vi "PWRVT.vi"() -> ()   [LabVIEW 2017]
uses:
  FcutionVI/Modbus function.ctl
  dll/LabVIEW_CSLib.dll
  dll/Modbus.dll
panel:
  in  "Data type":enum16{"Raw", "OA"}(ring)
  out "SN":string
  out "Acc RMS":u16[](array[numeric])
  out "Stop Time":timestamp
  in  "stop":bool
  out "Waveform Chart":dbl[][](graph)=[[0.0015869140625, -0.000732421875, -0.001220703125], [0.0008544921875, -0.0009765625, 0.000244140625], [0.0006103515625, -0.001220703125, 0.001220703125], [0.0015869140625, -0.0006103515625, 0.00048828125], [0.001953125, 0.0, -0.00048828125], [0.0009765625, 0.0, -0.000732421875], [0.0010986328125, -0.000244140625, -0.0006103515625], [0.0020751953125, 0.000244140625, 0.0], [0.002197265625, 0.001220703125, 0.0006103515625], [0.0020751953125, 0.0009765625, -0.000244140625], [0.0020751953125, 0.0, -0.0018310546875], [0.0013427734375, 0.0, -0.001708984375], [0.00048828125, 0.0001220703125, -0.0008544921875], [0.0009765625, -0.000244140625, -0.0010986328125], [0.0009765625, -0.0008544921875, -0.00146484375], [-0.0003662109375, -0.0003662109375, -0.0003662109375], [-0.0010986328125, 0.0, 0.0001220703125], [-0.0003662109375, -0.000244140625, -0.0008544921875], [-0.0006103515625, -0.000244140625, -0.001708984375], [-0.00146484375, 0.0010986328125, 0.0], [-0.000732421875, 0.001953125, 0.002685546875], [0.000244140625, 0.0010986328125, 0.0037841796875], [0.0, 0.0003662109375, 0.002197265625], [-0.0006103515625, 0.0006103515625, -0.0006103515625]]
  out "Modbus Function":T1
  out "Data Length 抓資料後的剩餘長度":u16(graph)
  in  "DAQ Interval (ms)":u32
  in  "SlaveID":u8=1
  out "error out":errorcluster
  in  "stopBits":i32(ring)=1 items=["None", "One", "Two", "OnePointFive"]
  in  "dataBits":i32=8
  in  "parity":i32(ring) items=["None", "Odd", "Even", "Mark", "Space"]
  in  "baudRate":i32=3000000
  in  "VISA resource name":refnum<visa-resource-name>
  # "x"
  # "y"
  # "z"
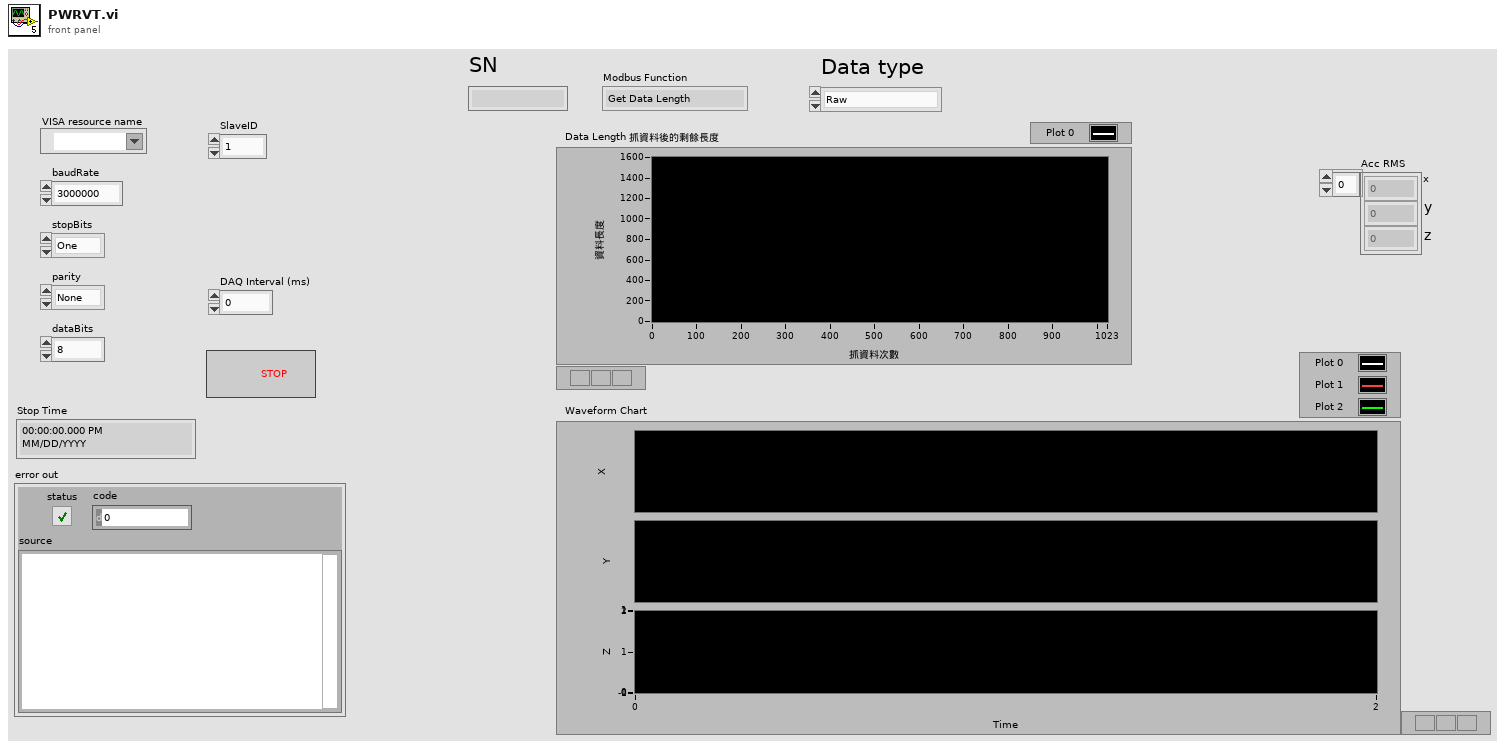
[diagram p1: front panel]
types:
  T1 = typedef "Modbus function.ctl" = enum16{"Get Data Length", "Normal Mode", "Bulk Mode"}
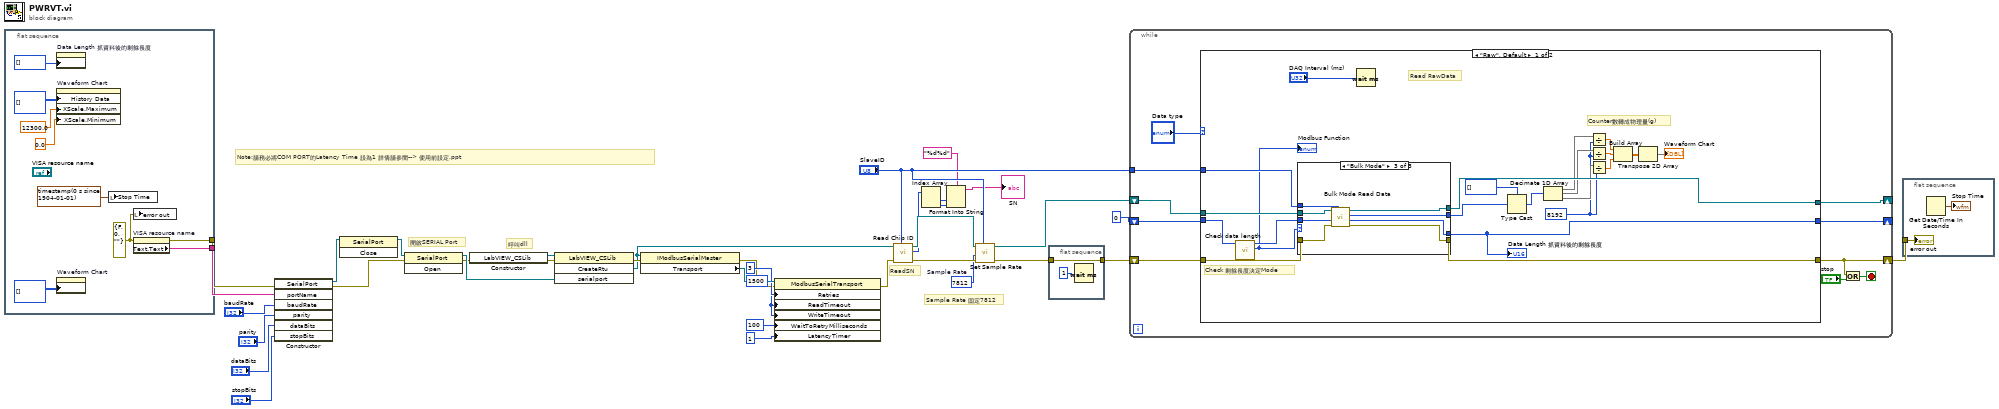
[diagram p0: block diagram]
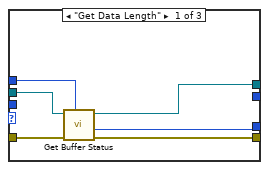
[diagram p2: hidden frame]
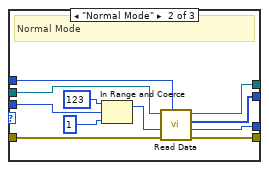
[diagram p3: hidden frame]
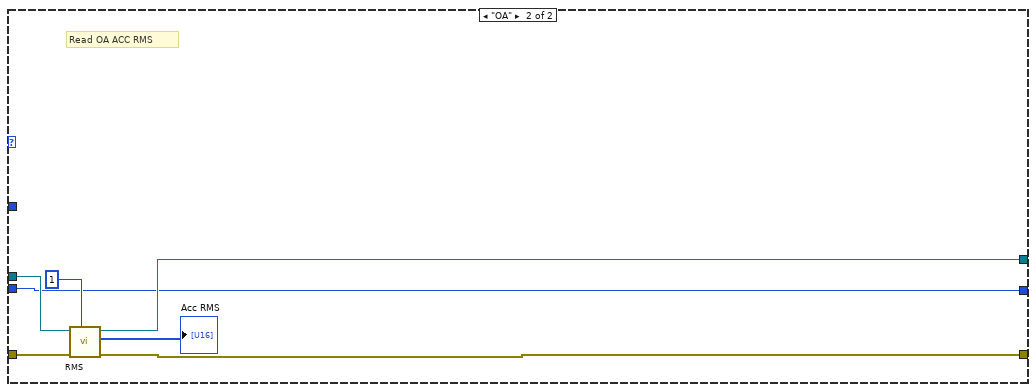
[diagram p4: hidden frame]
diagram:
  w1 = u16 7812  # Sample Rate
  w19 = 1500 ("ReadTimeout")
  # "Note:請務必將COM PORT的Latency Time 設為1 詳情請參閱--> 使用前設定.ppt"
  # "呼叫dll"
  # "開啟SERIAL Port"
  # "ReadSN"
  # "Sample Rate 固定7812"
  n1 = flat-sequence {
    tunnel: [w45] -> w36
    tunnel: [w44] -> w35
    frame #0 {
      w42 = errorcluster {"status"=FALSE, "code"=0, "source"=""} ("error constant")
      n2 = property on="Data Length 抓資料後的剩餘長度" class="WFChart (strict)"("History Data"=u16[] []) -> ()  [unwired: 2 in, 2 out]
      n3 = property on="Waveform Chart" class="WFChart (strict)"("History Data"=i16[][] [], "XScale.Maximum"=12300.0 ("X Scale.Range:Maximum"), "XScale.Minimum"=0.0 ("X Scale.Range:Minimum")) -> ()  [unwired: 2 in, 2 out]
      n4 = property on="Waveform Chart" class="WFChart (strict)"("History Data"=i16[][] []) -> ()  [unwired: 2 in, 2 out]
      n5 = local write "Stop Time"(timestamp(0 s since 1904-01-01) ("Stop Time")) -> ()
      n6 = local write "error out"(w42) -> ()
      n7 = property on="VISA resource name" class="VISAName"(error in=w42) -> (error out=w44:errorcluster, "Text.Text"=w45:string)  [unwired: 1 in, 1 out]
    }
  }
  n8 = constructor class="SerialPort"(error in=w35, "portName"=w36, "baudRate"="baudRate", "parity"="parity", "dataBits"="dataBits", "stopBits"="stopBits") -> (reference out=w27:refnum<k24>, error out=w11:errorcluster)  [unwired: 2 in, 6 out]
  n9 = invoke class="SerialPort" method="Close"(reference=w27) -> (reference out=w26:refnum<k24>)  [unwired: 2 in, 2 out]
  n10 = invoke class="SerialPort" method="Open"(reference=w26, error in=w11) -> (reference out=w30:refnum<k24>, error out=w29:errorcluster)  [unwired: 1 in, 1 out]
  n11 = constructor class="LabVIEW_CSLib"(error in=w29) -> (reference out=w24:refnum<k24>, error out=w28:errorcluster)  [unwired: 2 in, 1 out]
  n12 = invoke class="LabVIEW_CSLib" method="CreateRtu"(reference=w24, error in=w28, "serialport"=w30) -> (error out=w17:errorcluster, "CreateRtu"=w13:refnum<k24>)  [unwired: 1 in, 2 out]
  n13 = property class="IModbusSerialMaster"(reference=w13, error in=w17) -> (error out=w16:errorcluster, "Transport"=w21:refnum<k24>)  [unwired: 1 out]
  n14 = property class="ModbusSerialTransport"(reference=w21, error in=w16, "Retries"=3, "ReadTimeout"=w19, "WriteTimeout"=w19, "WaitToRetryMilliseconds"=100, "LatencyTimer"=1) -> (error out=w9:errorcluster)  [unwired: 1 out]
  n15 = call "Read Chip ID.vi"("SlaveID"="SlaveID", "error in (no error)"=w9, ".NET Refnum in"=w13) -> ("error out"=w12:errorcluster, "32bit integer"=w6:i32[], ".NET Refnum out"=w10:refnum<k24>)  [unwired: 6 in]
  n16 = Index Array(array=w6) -> (element #1=w5:i32, element #2=w4:i32)  [unwired: 2 in]
  n17 = Format Into String(format string="%d%d", w5, w4) -> (resulting string=→"SN":string)  [unwired: 2 in, 1 out]
  n18 = call "Set Sample Rate.vi"("SlaveID"="SlaveID", "error in (no error)"=w12, "Sample Rate"=w1, ".NET Refnum in"=w10) -> ("error out"=w25:errorcluster, ".NET Refnum out"=w8:refnum<k24>)  [unwired: 6 in]
  n19 = flat-sequence {
    tunnel: w25 -> [w46]
    tunnel: [w46] -> w7
    frame #0 {
      n20 = Wait (ms)(milliseconds to wait=u32 1) -> ()  [unwired: 1 out]
    }
  }
  n21 = while {
    shift-right: [w51] -> w23
    shift-left: w7 -> [w56]
    shift-right: [w49] -> _
    shift-left: u16 0 ("# samples in buffer") -> [w54]
    shift-right: [w50] -> _
    shift-left: w8 -> [w57]
    tunnel: "SlaveID" -> [w55]
    stop <- w52 stop-if-true
    n22 = case shown="\"Raw\", Default" "Data type" {
      tunnel: w57 -> [w79 w111]
      tunnel: w56 -> [w78 w108]
      tunnel: w55 -> [w76 _]
      tunnel: w54 -> [w75 w106]
      tunnel: [w70 w107] -> w51
      tunnel: [w69 w110] -> w50
      tunnel: [w68 w106] -> w49
      frame "Raw", Default {
        w63 = 8192 ("length")
        # "Counter數轉成物理量(g)"
        # "Check 剩餘長度決定Mode"
        # "Read RawData"
        n23 = call "Check data length.vi"("# samples in buffer"=w75) -> ("Modbus Function"=w73:T1, "# samples in buffer out"=w74:u16)  [unwired: 9 in]
        "Modbus Function" <- w73
        n24 = case shown="\"Bulk Mode\"" w73 {
          tunnel: w79 -> [w85 w96 w104]
          tunnel: [w84 w87 w101] -> w68
          tunnel: [w83 w93 w102] -> w70
          tunnel: w74 -> [_ w91 w98]
          tunnel: w76 -> [w82 w90 w99]
          tunnel: [w81 w89 w100] -> w69
          tunnel: w78 -> [w80 w88 w103]
          tunnel: [_ w86 w97] -> w71
          frame "Get Data Length" {
            n25 = call "Get Buffer Status.vi"("SlaveID"=w82, "error in (no error)"=w80, ".NET Refnum in"=w85) -> ("error out"=w83:errorcluster, "# samples in buffer"=w84:u16, ".NET Refnum out"=w81:refnum<k24>)  [unwired: 5 in, 1 out]
          }
          frame "Normal Mode" {
            # "Normal Mode"
            n26 = In Range and Coerce(upper limit=u16 123, x=w91, lower limit=u16 1) -> (coerced(x)=w92:u16)  [unwired: 1 out]
            n27 = call "Read Data.vi"("SlaveID"=w90, "error in (no error)"=w88, "# samples to read"=w92, ".NET Refnum in"=w96) -> ("error out"=w93:errorcluster, "# samples in buffer"=w87:u16, "Vib"=w86:u16[], "reference out"=w89:refnum<k24>)  [unwired: 4 in]
          }
          frame "Bulk Mode" {
            n28 = call "Bulk Mode Read Data.vi"("SlaveID"=w99, "error in (no error)"=w103, "# samples to read"=w98, ".NET Refnum in"=w104) -> ("error out"=w102:errorcluster, "# samples in buffer"=w101:u16, "Vib"=w97:u16[], "reference out"=w100:refnum<k24>)  [unwired: 4 in]
          }
        }
        "Data Length 抓資料後的剩餘長度" <- w68
        n29 = Wait (ms)(milliseconds to wait="DAQ Interval (ms)") -> ()  [unwired: 1 out]
        n30 = Type Cast(type=i16[] [], x=w71) -> (*(type *) &x=w67:i16[])
        n31 = Decimate 1D Array(w67) -> (w64:i16[], w65:i16[], w66:i16[])
        n32 = Divide(x=w64, y=w63) -> (x/y=w61:dbl[])
        n33 = Divide(x=w65, y=w63) -> (x/y=w60:dbl[])
        n34 = Divide(x=w66, y=w63) -> (x/y=w59:dbl[])
        n35 = Build Array(w61, w60, w59) -> (w58:dbl[][])
        n36 = Transpose 2D Array(2D array=w58) -> (transposed array=→"Waveform Chart":dbl[][])
      }
      frame "OA" {
        # "Read OA ACC RMS"
        n37 = call "RMS.vi"("SlaveID"=u8 1, "error in (no error)"=w108, ".NET Refnum in"=w111) -> ("error out"=w107:errorcluster, "Acc RMS"=→"Acc RMS":u16[], "reference out"=w110:refnum<k24>)  [unwired: 6 in]
      }
    }
    n38 = Or(x=w51, y="stop") -> (x .or. y?=w52:bool)
  }
  n39 = flat-sequence {
    tunnel: w23 -> [w112]
    frame #0 {
      n40 = Get Date/Time In Seconds() -> (seconds since 1Jan1904=→"Stop Time":timestamp)
      "error out" <- w112
    }
  }
